vi "validate line configuration.vi"(7 "Module Config":refnum<class "Increment configuration.lvclass">, 11 "Mappings in":T1) -> (1 "valid?":bool, 2 "errors":string, 3 "Mappings out":T1)   [LabVIEW 2015, in "Increment editor node.lvclass"]
doc: "This VI validates modifications to the table of lines and returns any errors as strings."
uses:
  Increment editor node.lvclass
  Mappings.ctl
  <vilib>/NI/Tag Bus Module Framework/channel/TBM channel.lvclass
  module/configuration/Line.ctl
  Map.ctl
  module/configuration/Increment configuration.lvclass
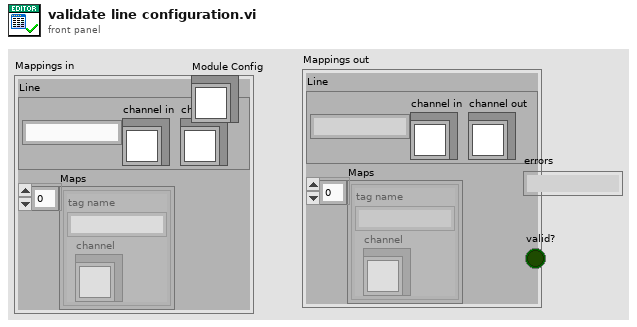
[diagram p1: front panel]
types:
  T1 = typedef "Increment editor node.lvclass/Mappings.ctl" = cluster{"Line":T2, "Maps":T3[]}
  T2 = typedef "Increment configuration.lvclass/Line.ctl" = cluster{"Name":string, "channel in":refnum<class "TBM channel.lvclass">, "channel out":refnum<class "TBM channel.lvclass">}
  T3 = typedef "Increment editor node.lvclass/Map.ctl" = cluster{"channel":refnum<class "TBM channel.lvclass">, "tag name":string}
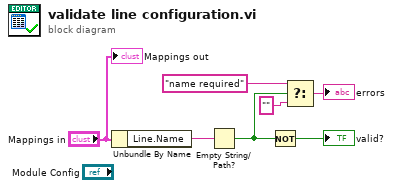
[diagram p0: block diagram]
diagram:
  n1 = Unbundle By Name("Mappings in") -> ("Line.Name"=w1:string)
  n2 = Empty String/Path?(string/path=w1) -> (empty?=w5:bool)
  n3 = Not(x=w5) -> (.not. x?=→"valid?":bool)
  n4 = Select(t="name required", s=w5, f="") -> (s? t:f=→"errors":string)
  "Mappings out" <- "Mappings in"
